vi "Unsubscribe.vi"(7 "Unique Subscriber ID":string, 8 "error in (no error)":errorcluster, 10 "Subscription Name":string, 11 "ISubject in":refnum<class "ISubject.lvclass">) -> (0 "error out":errorcluster, 3 "ISubject out":refnum<class "ISubject.lvclass">)   [LabVIEW 2015, in "Observer.lvlib" / "ISubject.lvclass"]
uses:
  ISubject.lvclass
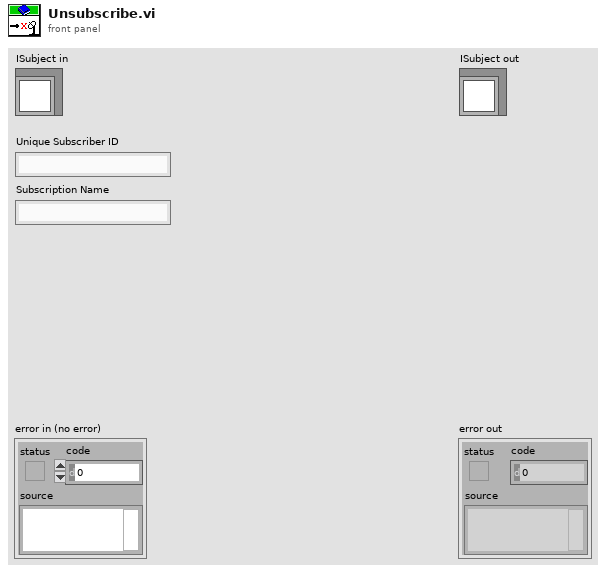
[diagram p1: front panel]
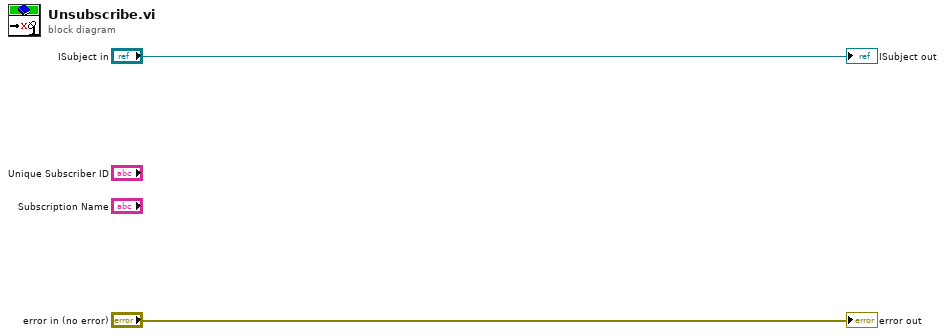
[diagram p0: block diagram]
diagram:
  "error out" <- "error in (no error)"
  "ISubject out" <- "ISubject in"
